vi "addNewElement.vi"(6 "firstItem? (F)":bool, 8 "error in (no error)":errorcluster, 9 "prevObjRef":refnum<vi>, 10 "clusterInfo.reference":refnum<vi>, 11 "UnsignedLongLong in":refnum<class "UnsignedLongLong.lvclass">) -> (0 "error out":errorcluster, 3 "UnsignedLongLong out":refnum<class "UnsignedLongLong.lvclass">)   [LabVIEW 2016, in "UnsignedLongLong.lvclass"]
uses:
  UnsignedLongLong.lvclass
  D:/Code/ts_SALLabVIEW/SALTypeGenerator/Elements/Numeric/Numeric.lvclass
  <vilib>/numeric/LVNumericRepresentation.ctl
  Numeric/Numeric.lvclass/Numeric.ctl
  Unsigned/Unsigned.lvclass
  Numeric/Numeric.lvclass
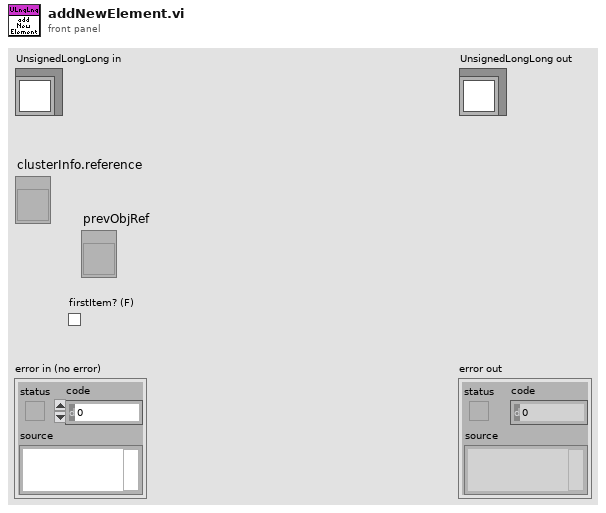
[diagram p1: front panel]
types:
  T1 = typedef "LVNumericRepresentation.ctl" = enum32{"Extended Precision", "Double Precision", "Single Precision", "Long", "Word", "Byte", "Unsigned Long", "Unsigned Word", "Unsigned Byte", "Complex Extended", "Complex Double", "Complex Single", "Quad", "Unsigned Quad", "Fixed-Point"}
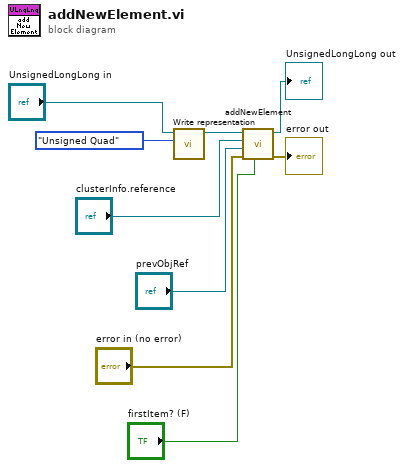
[diagram p0: block diagram]
diagram:
  n1 = call "Write representation.vi"("Numeric Representation"=LVNumericRepresentation."Unsigned Quad", "Numeric in"="UnsignedLongLong in") -> ("Numeric out"=w2:refnum<class "UnsignedLongLong.lvclass">)  [unwired: 9 in]
  n2 = call-parent "addNewElement.vi"("firstItem? (F)"="firstItem? (F)", "error in (no error)"="error in (no error)", "prevObjRef"="prevObjRef", "clusterInfo.reference"="clusterInfo.reference", "Numeric in"=w2) -> ("error out"=→"error out":errorcluster, "Numeric out"=→"UnsignedLongLong out":refnum<class "UnsignedLongLong.lvclass">)  [unwired: 5 in]
